vi "BoolCmd_Multiplexor_Array.vi"(9 "Ready":bool=TRUE, 10 "Command Cancel":bool, 11 "Commands":bool[](array[boolean])) -> (1 "Do Cancel":bool[](array[boolean]), 3 "Do Command":bool[](array[boolean]))   [LabVIEW 2019, in "Trajectory_Library.lvlib"]
uses:
  Trajectory_Library.lvlib
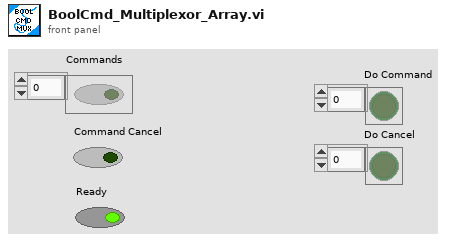
[diagram p1: front panel]
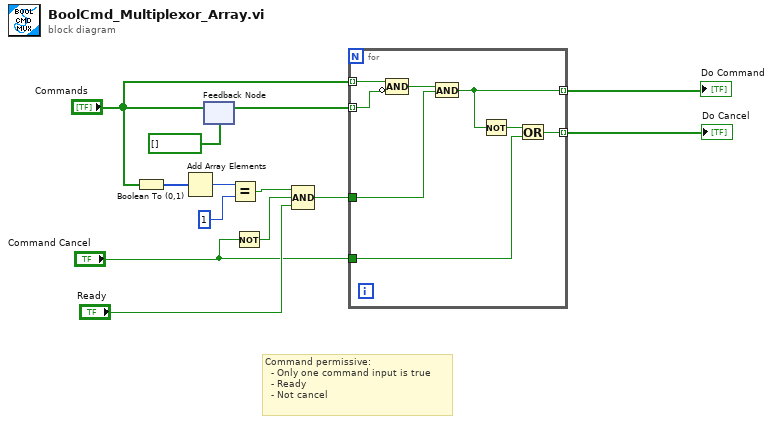
[diagram p0: block diagram]
diagram:
  # "Command permissive:\n  - Only one command input is true\n  - Ready\n  - Not cancel"
  n1 = Boolean To (0,1)(Boolean="Commands") -> (0, 1=w13:i16[])
  n2 = Add Array Elements(numeric array=w13) -> (sum=w12:i16)
  n3 = feedback-in #1("Commands") -> ()
  n4 = feedback #1(bool[] [] ("Command 1")) -> (w8:bool[])
  n5 = Equal?(x=w12, y=i16 1) -> (x = y?=w7:bool)
  n6 = Not(x="Command Cancel") -> (.not. x?=w6:bool)
  n7 = Compound Arithmetic op=AND(w7, w6, "Ready") -> (w4:bool)
  n8 = for {
    tunnel: "Commands" -> [w21] mode=indexing
    tunnel: w8 -> [w20] mode=indexing
    tunnel: w4 -> [w18]
    tunnel: [w17] -> w3 mode=indexing
    tunnel: "Command Cancel" -> [w15]
    tunnel: [w14] -> w1 mode=indexing
    n9 = Compound Arithmetic op=AND(w21, invert w20) -> (w19:bool)
    n10 = And(x=w19, y=w18) -> (x .and. y?=w17:bool)
    n11 = Not(x=w17) -> (.not. x?=w16:bool)
    n12 = Or(x=w16, y=w15) -> (x .or. y?=w14:bool)
  }
  "Do Command" <- w3
  "Do Cancel" <- w1
